vi "Charging_Measure VBAT.vi"(8 "error in":errorcluster) -> (0 "error out":errorcluster, 2 "VBAT (volts)":dbl=nan format="%.4f", 3 "ADC Counts":dbl=nan)   [LabVIEW 2010]
doc: "This function reads the IPG VBAT ADC count and converts it to volts.\n\nThe IPG VBAT ADC is 12-bit unsigned, full scale is 5.00 volts.\nThe ADC scale factor is 0.001221001 per ADC bit. (4095 * 0.001221001 = 5.0000 volts)"
uses:
  Telemetry/Typedef Command List.ctl
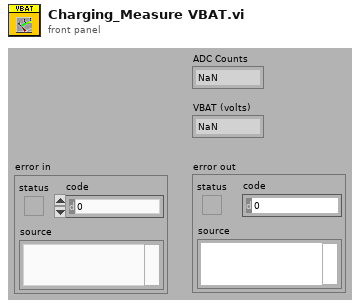
[diagram p1: front panel]
types:
  T1 = typedef "Typedef Command List.ctl" = enum16{"Get xPG Status", "xPG Stimulation", "Select Program", "Increment Program Amplitude", "Decrement Program Amplitude", "Get PoP Constants", "Get PPC Constants", "Get Program Names", "Set Pulse Amplitude", "Increment Pulse Amplitude", "Decrement Pulse Amplitude", "Get Pulse Widths", "Set Pulse Widths", "Increment Pulse Width", "Decrement Pulse Width", "Get Program Frequency", "Set Program Frequency", "Increment Program Frequency", "Decrement Program Frequency", "Inject Event", "Charging Control", "Get xPG Identity", "Set xPG Identity", "Restore Program Defaults", "Get Program Definition", "Set Program Definition", "Get Program Constants", "Set Program Constants", "Get Configurable Device Parameters", "Set Configurable Device Parameters", "Get Pulse Constants", "Set Pulse Constants", "Get Lead Limits", "Set Lead Limits", "Get Channel Calibrations", "Set Channel Calibrations", "<reserved 2>", "<reserved 3>", "<reserved 4>", "<reserved 5>", "<reserved 6>", "<reserved 7>", "Get Stim Asic HV Calibrations", "Set Stim Asic HV Calibrations", "<reserved 8>", "<reserved 9>", "Get CP Data", "Set CP Data", "Clear Log", "Read Log", "Append Log", "Get Patient Program Runtime", "Set Patient Program Runtime", "Impedance Measurement", "Enter Storage Mode", "Echo Short", "Echo Long", "Get General Calibration", "Set General Calibration", "Get Trim List", "Set Trim List", "Get Counter", "Set Counter", "Get Test Stimulation", "Set Test Stimulation", "Get Titration Stimulation", "Set Titration Stimulation", "Get Ramp Time", "Set Ramp Time", "Get VBAT", "Set Software Description Block", "Get Software Description Block", "Write Memory", "Read Memory", "Reset xPG", "Erase Flash Block", "Write Vectors", "Read Vectors", "Diagnostic Data", "Set Background Impedance", "Get Background Impedence ", "Set Test Waveform", "Calibrate Channel", "Get Log Range", "Reserved 0x55", "Reserved 0x56", "MICS Options", "Pair PPC", "Pair POP", "Stop Bootloader", "Tune MICS", "MICS Diagnostics", "Undefined"}
  T2 = cluster{"Command":T1, "Function":enum16{"Open Session", "Close Session", "Downlink Only", "Uplink Only", "Transceive (DN -> UP)"}, "MICS_ID":u32, "EXID":u32, "Use Local":bool, "Transceive Delay mS":dbl, "CP_DATA IN":u8[], "Parameters":string}
  T3 = cluster{"Response Token":string, "Response Code":string, "bChecksum Valid":bool, "tChecksum Valid":bool, "CP_DATA OUT":u8[], "Data":string}
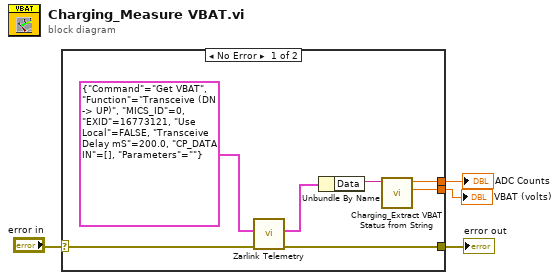
[diagram p0: block diagram]
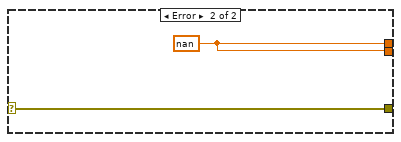
[diagram p2: hidden frame]
diagram:
  n1 = case shown="No Error" "error in" {
    selector: "error in" -> [w11 w13]
    tunnel: [w10 w13] -> w3
    tunnel: [w6 w12] -> w1
    tunnel: [w5 w12] -> w2
    frame No Error {
      n2 = call "Zarlink Telemetry.vi"("error in (no error)"=w11, "Input"=T2 {"Command"=enum."Get VBAT", "Function"=enum."Transceive (DN -> UP)", "MICS_ID"=0, "EXID"=16773121, "Use Local"=FALSE, "Transceive Delay mS"=200.0, "CP_DATA IN"=[], "Parameters"=""}) -> ("error out"=w10:errorcluster, "Output"=w8:T3)  [unwired: 7 in, 1 out]
      n3 = Unbundle By Name(w8) -> ("Data"=w7:string)
      n4 = call "Charging_Extract VBAT Status from String.vi"("Get VBAT String"=w7) -> ("VBAT (volts)"=w6:dbl, "ADC Counts"=w5:dbl)  [unwired: 9 in]
    }
    frame Error {
      w12 = nan ("ADC Counts")
    }
  }
  "error out" <- w3
  "ADC Counts" <- w2
  "VBAT (volts)" <- w1
